vi "Convert IMAQ to LV Image.vi"(8 "error in (no error)":errorcluster, 11 "IMAQImage In (RGB 32)":T2) -> (0 "error out":errorcluster, 2 "Output Image":T1, 3 "IMAQImage Out":T2)   [LabVIEW 2013]
doc: "This VI converts an RGB32 IMAQ image to a LabVIEW image."
uses:
  <vilib>/vision/Image Controls.llb/IMAQ Image.ctl
  <vilib>/picture/picture.llb/imagedata.ctl
  <resource>/objmgr/IMAQImage.rc
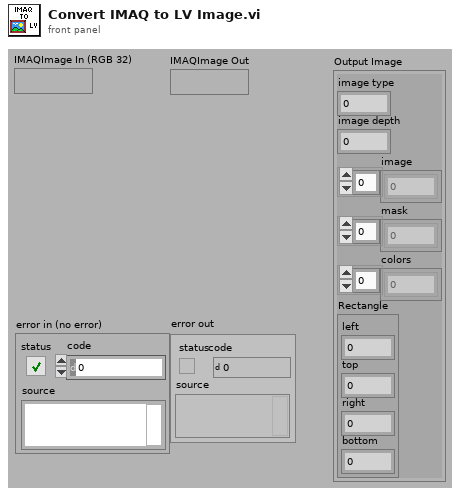
[diagram p1: front panel]
types:
  T1 = typedef "imagedata.ctl" = cluster{"image type":i32, "image depth":i32, "image":u8[], "mask":u8[], "colors":u32[], "Rectangle":cluster{"left":i16, "top":i16, "right":i16, "bottom":i16}}
  T2 = typedef "IMAQ Image.ctl" = refnum<image>
  T3 = typedef "Image Type" = u32
  T4 = cluster{"left":i16, "top":i16, "right":i16, "bottom":i16}
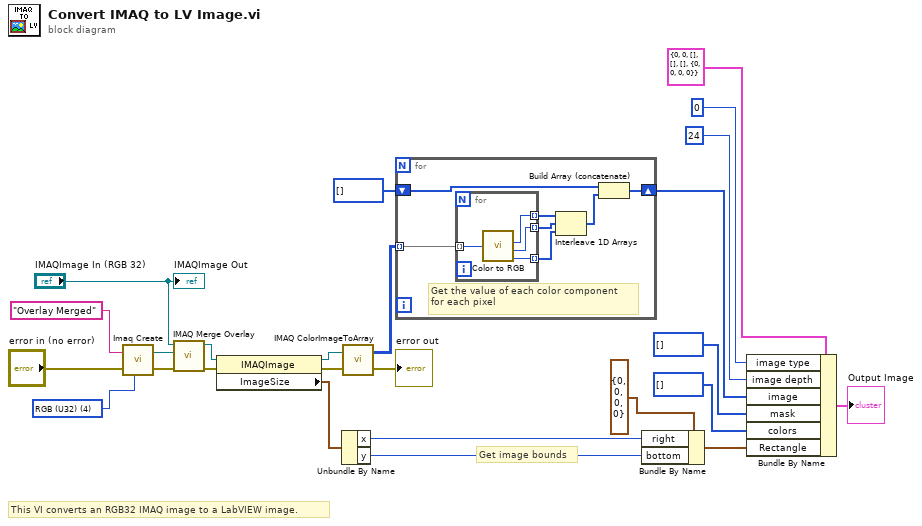
[diagram p0: block diagram]
diagram:
  w5 = T3 4 items=["Grayscale (U8)", "Grayscale (I16)", "Grayscale (SGL)", "Complex (CSG)", "RGB (U32)", "HSL (U32)", "RGB (U64)", "Grayscale (U16)"] ("Image Type")
  # "This VI converts an RGB32 IMAQ image to a LabVIEW image."
  # "Get image bounds"
  n1 = call "Imaq Create"("Image Name"="Overlay Merged", "Image Type"=w5, "error in (no error)"="error in (no error)") -> ("New Image"=w7:T2, "error out"=w3:errorcluster)  [unwired: 2 in]
  n2 = call "IMAQ Merge Overlay"("error in (no error)"=w3, "Image Dst"=w7, "Image Src"="IMAQImage In (RGB 32)") -> ("error out"=w2:errorcluster, "Image Dst Out"=w9:T2)  [unwired: 7 in]
  n3 = property class="IMAQImage"(reference=w9, error in=w2) -> (reference out=w1:T2, error out=w15:errorcluster, "ImageSize"=w24:cluster{"x":i32, "y":i32})
  n4 = Unbundle By Name(w24) -> ("x"=w20:i32, "y"=w19:i32)
  n5 = call "IMAQ ColorImageToArray"("Image"=w1, "error in (no error)"=w15) -> ("Image Pixels (U32)"=w12:u32[][], "error out"=→"error out":errorcluster)  [unwired: 2 in, 1 out]
  n6 = for {
    shift-right: [w30] -> w17
    shift-left: u8[] [] -> [w31]
    tunnel: w12 -> [w29] mode=indexing
    # "Get the value of each color component\nfor each pixel"
    n7 = for {
      tunnel: w29 -> [w36] mode=indexing
      tunnel: [w35] -> w28 mode=indexing
      tunnel: [w34] -> w27 mode=indexing
      tunnel: [w33] -> w26 mode=indexing
      n8 = call <vilib>:"Color to RGB.vi"("Color"=w36) -> ("R"=w35:u8, "G"=w34:u8, "B"=w33:u8)  [unwired: 1 out]
    }
    n9 = Interleave 1D Arrays(w28, w27, w26) -> (w32:u8[])
    n10 = Build Array (concatenate)(w31, w32) -> (w30:u8[])
  }
  n11 = Bundle By Name(cluster=T4 {"left"=0, "top"=0, "right"=0, "bottom"=0} ("Rectangle"), "right"=w20, "bottom"=w19) -> (w23:T4)
  n12 = Bundle By Name(cluster=T1 {"image type"=0, "image depth"=0, "image"=[], "mask"=[], "colors"=[], "Rectangle"={"left"=0, "top"=0, "right"=0, "bottom"=0}} ("Image Data"), "image type"=0, "image depth"=24 ("Bit Depth (0)"), "image"=w17, "mask"=u8[] [], "colors"=u32[] [], "Rectangle"=w23) -> (→"Output Image":T1)
  "IMAQImage Out" <- "IMAQImage In (RGB 32)"
